vi "HandleErrorStates.vi"(8 "error in (no error)":errorcluster) -> (0 "error out":errorcluster, 3 "Enum":T1)   [LabVIEW 2018, in "feGEM DataPacker.lvlib"]
uses:
  StateMachineTypeDef.ctl
  feGEM DataPacker.lvlib
  ErrorTypes.ctl
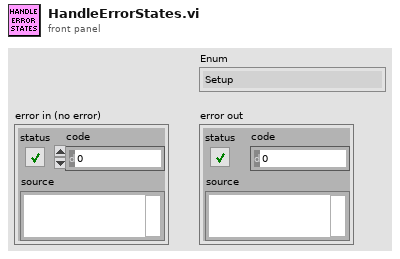
[diagram p1: front panel]
types:
  T1 = typedef "feGEM DataPacker.lvlib/StateMachineTypeDef.ctl" = enum16{"Setup", "Setup SSH", "Connect To Midas", "Get And Set Event Size", "Re-initialise", "Update status", "BundleDataInQueue", "SerializeBundle", "SendData", "Shutdown", "HandleErrorStates", "Wait"}
  T2 = typedef "feGEM DataPacker.lvlib/ErrorTypes.ctl" = i32
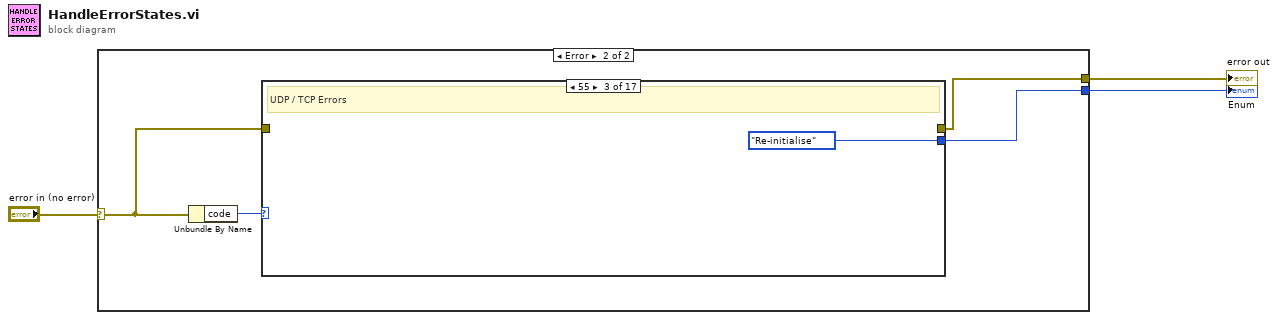
[diagram p0: block diagram]
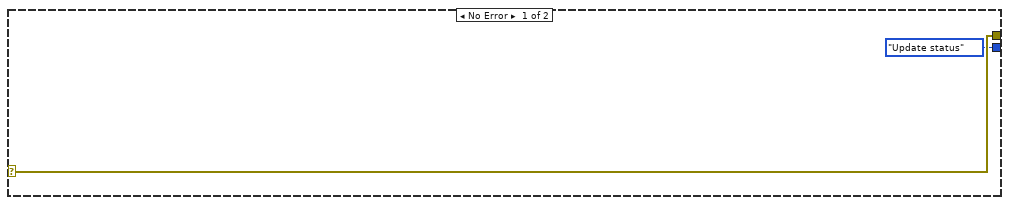
[diagram p2: hidden frame]
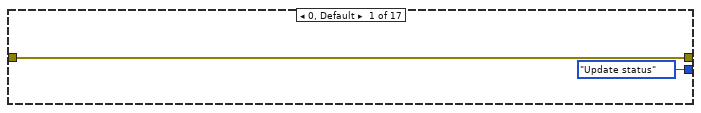
[diagram p3: hidden frame]
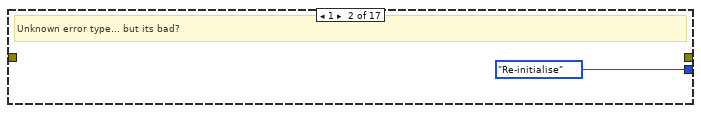
[diagram p4: hidden frame]
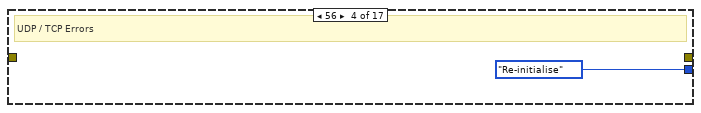
[diagram p5: hidden frame]
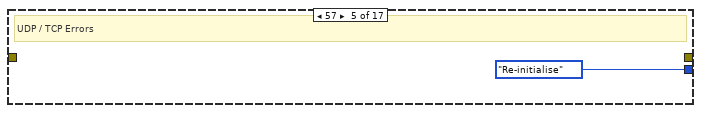
[diagram p6: hidden frame]
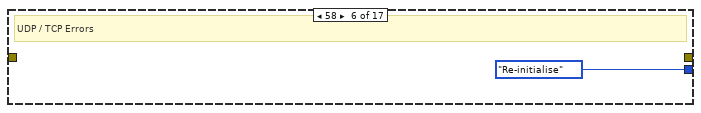
[diagram p7: hidden frame]
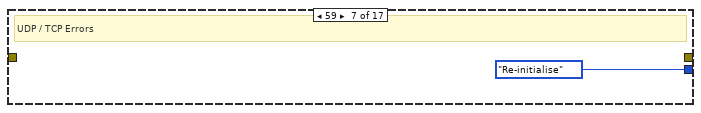
[diagram p8: hidden frame]
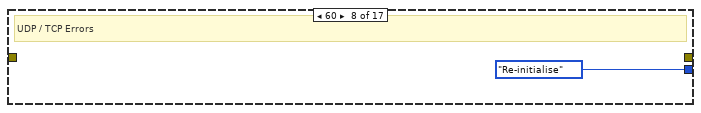
[diagram p9: hidden frame]
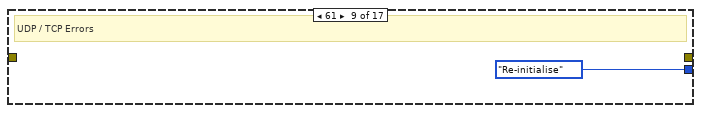
[diagram p10: hidden frame]
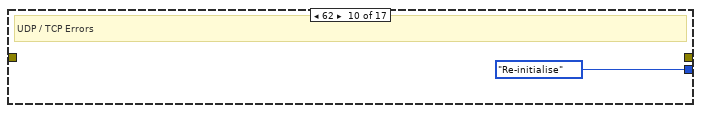
[diagram p11: hidden frame]
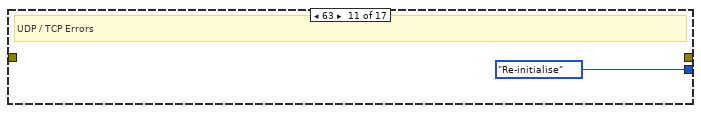
[diagram p12: hidden frame]
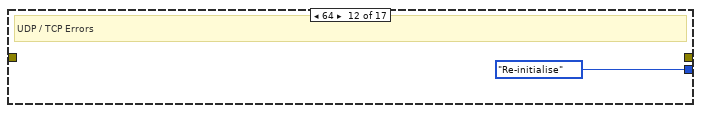
[diagram p13: hidden frame]
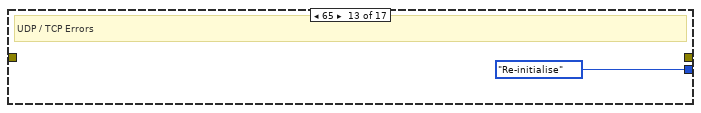
[diagram p14: hidden frame]
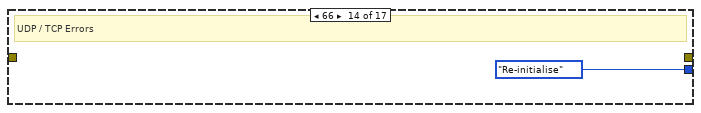
[diagram p15: hidden frame]
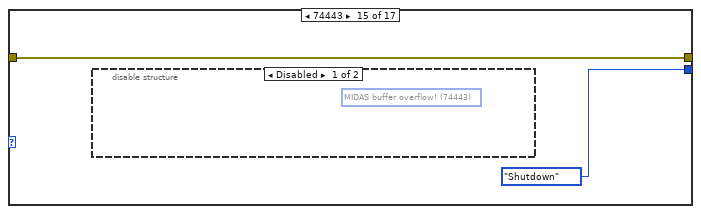
[diagram p16: hidden frame]
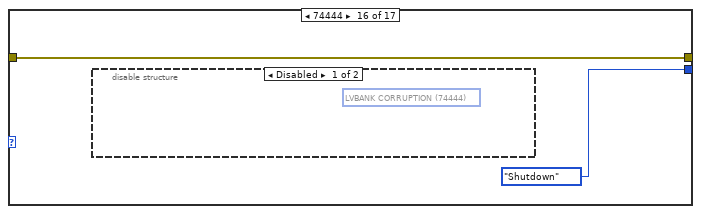
[diagram p18: hidden frame]
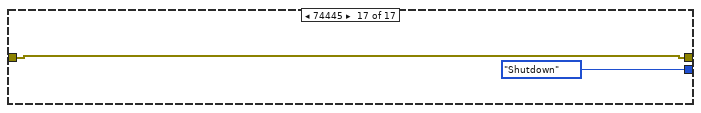
[diagram p20: hidden frame]
diagram:
  n1 = case shown="Error" "error in (no error)" {
    selector: "error in (no error)" -> [w5 w6]
    tunnel: [StateMachineTypeDef."Update status" ("Enum") w8] -> w2
    tunnel: [w5 w7] -> w3
    frame No Error {
    }
    frame Error {
      n2 = Unbundle By Name(w6) -> ("code"=w9:i32)
      n3 = case shown="55" w9 {
        tunnel: [StateMachineTypeDef."Update status" ("Enum") StateMachineTypeDef."Re-initialise" ("Enum") StateMachineTypeDef."Re-initialise" ("Enum") StateMachineTypeDef."Re-initialise" ("Enum") StateMachineTypeDef."Re-initialise" ("Enum") StateMachineTypeDef."Re-initialise" ("Enum") StateMachineTypeDef."Re-initialise" ("Enum") StateMachineTypeDef."Re-initialise" ("Enum") StateMachineTypeDef."Re-initialise" ("Enum") StateMachineTypeDef."Re-initialise" ("Enum") StateMachineTypeDef."Re-initialise" ("Enum") StateMachineTypeDef."Re-initialise" ("Enum") StateMachineTypeDef."Re-initialise" ("Enum") StateMachineTypeDef."Re-initialise" ("Enum") StateMachineTypeDef."Shutdown" ("Enum") StateMachineTypeDef."Shutdown" ("Enum") StateMachineTypeDef."Shutdown" ("Enum")] -> w8
        tunnel: [w11 _ _ _ _ _ _ _ _ _ _ _ _ _ w25 w27 w30] -> w7
        tunnel: w6 -> [w11 _ _ _ _ _ _ _ _ _ _ _ _ _ w25 w27 w30]
        frame 0, Default {
        }
        frame 1 {
          # "Unknown error type... but its bad?"
        }
        frame 55 {
          # "UDP / TCP Errors"
        }
        frame 56 {
          # "UDP / TCP Errors"
        }
        frame 57 {
          # "UDP / TCP Errors"
        }
        frame 58 {
          # "UDP / TCP Errors"
        }
        frame 59 {
          # "UDP / TCP Errors"
        }
        frame 60 {
          # "UDP / TCP Errors"
        }
        frame 61 {
          # "UDP / TCP Errors"
        }
        frame 62 {
          # "UDP / TCP Errors"
        }
        frame 63 {
          # "UDP / TCP Errors"
        }
        frame 64 {
          # "UDP / TCP Errors"
        }
        frame 65 {
          # "UDP / TCP Errors"
        }
        frame 66 {
          # "UDP / TCP Errors"
        }
        frame 74443 {
          n4 = disable-structure shown="Disabled" {
            frame Disabled {
              (unwired) T2 74443 items=["No Error"=0, "Network: mgNotSupported"=53, "Network: ncBadAddressErr"=54, "Network: ncInProgressErr"=55, "Network: ncTimeOutErr"=56, "Network: ncBusyErr"=57, "Network: ncNotSupportedErr"=58, "Network: ncNetErr"=59, "Network: ncAddrInUseErr"=60, "Network: ncSysOutOfMemErr"=61, "Network: ncSysOutOfMemErr"=62, "Network: ncConnRefusedErr"=63, "Network: ncAlreadyConnectedErr"=65, "Network: ncConnClosedErr"=66, "MIDAS buffer overflow!"=74443, "LVBANK CORRUPTION"=74444] ("Ring")
            }
            frame Enabled {
            }
          }
        }
        frame 74444 {
          n5 = disable-structure shown="Disabled" {
            frame Disabled {
              (unwired) T2 74444 items=["No Error"=0, "Network: mgNotSupported"=53, "Network: ncBadAddressErr"=54, "Network: ncInProgressErr"=55, "Network: ncTimeOutErr"=56, "Network: ncBusyErr"=57, "Network: ncNotSupportedErr"=58, "Network: ncNetErr"=59, "Network: ncAddrInUseErr"=60, "Network: ncSysOutOfMemErr"=61, "Network: ncSysOutOfMemErr"=62, "Network: ncConnRefusedErr"=63, "Network: ncAlreadyConnectedErr"=65, "Network: ncConnClosedErr"=66, "LVBANK CORRUPTION"=74444] ("Ring")
            }
            frame Enabled {
            }
          }
        }
        frame 74445 {
        }
      }
    }
  }
  "error out" <- w3
  "Enum" <- w2
